vi "Load Firmware Data.vi"(8 "Error In":errorcluster, 9 "Device Type":u16(ring) items=["chipKIT Uno32", "chipKIT uC32", "chipKIT Max32", "chipKIT DP32"], 10 "Device Family":u16(ring) items=["National Instruments", "Digilent", "Arduino"], 11 "Firmware Version":u16(ring) items=["LINX -  Serial / USB", "LINX -  Serial / USB [Debug] "]) -> (0 "Error Out":errorcluster, 2 "Firmware Interface":T1, 3 "Firmware ReadMe":string)   [LabVIEW 2013, in "LVH-LINX.lvlib"]
doc: "Load specified firmware readme."
uses:
  <vilib>/LabVIEW Hacker/LINX/LVH-LINX.lvlib
  <vilib>/LabVIEW Hacker/LINX/Private/Device/Type Defs/Firmware Interface.ctl
panel:
  in  "Device Family":u16(ring) items=["National Instruments", "Digilent", "Arduino"]
  in  "Device Type":u16(ring) items=["chipKIT Uno32", "chipKIT uC32", "chipKIT Max32", "chipKIT DP32"]
  in  "Firmware Version":u16(ring) items=["LINX -  Serial / USB", "LINX -  Serial / USB [Debug] "]
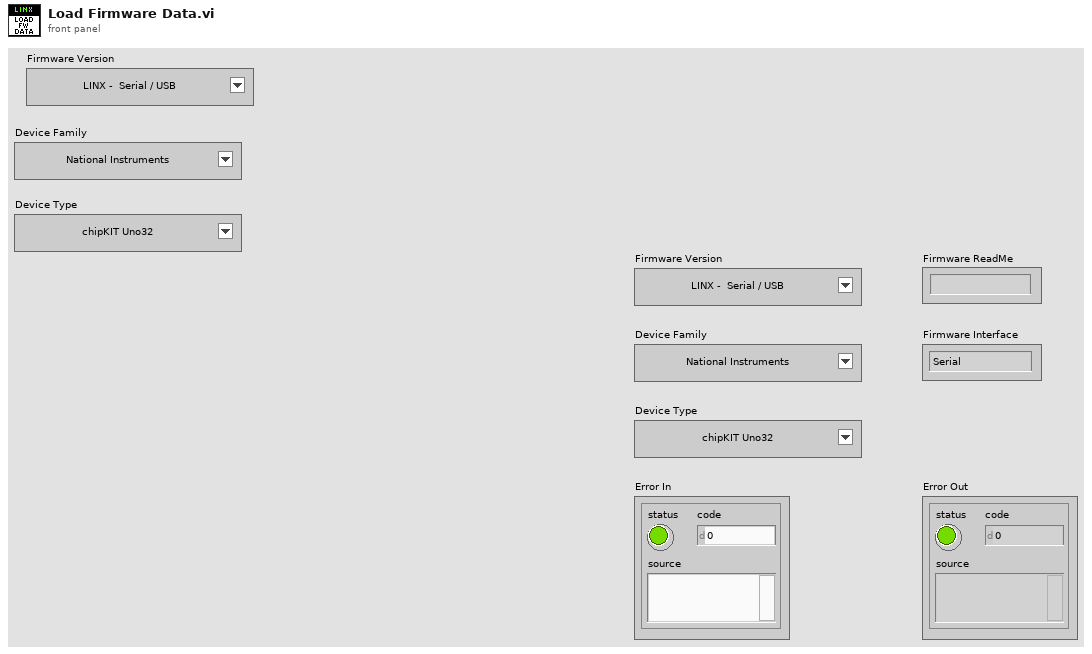
[diagram p1: front panel]
types:
  T1 = typedef "LVH-LINX.lvlib/Firmware Interface.ctl" = enum32{"Serial ", "Ethernet", "WIFI"}
  T2 = typedef "LVH-LINX.lvlib/Generic Device.ctl" = cluster{"DI Channels":u8[], "DO Channels":u8[], "AI":u8[], "AO":u8[], "PWM":u8[], "QE":u8[], "UART":u8[], "I2C 2":u8[], "SPI":u8[], "CAN":u8[], "AI Ref (V)":dbl, "Firmware Program Interfaces":enum16{"N/A", "Serial / USB", "USB", "TCP"}[], "Firmware Versions":T3[], "Name":string, "AO Resolution (Bits)":u8, "AO Ref (V)":dbl}
  T3 = typedef "LVH-LINX.lvlib/Firmware Version.ctl" = cluster{"Name":string, "Relative Path":string, "Firmware Interface":T1}
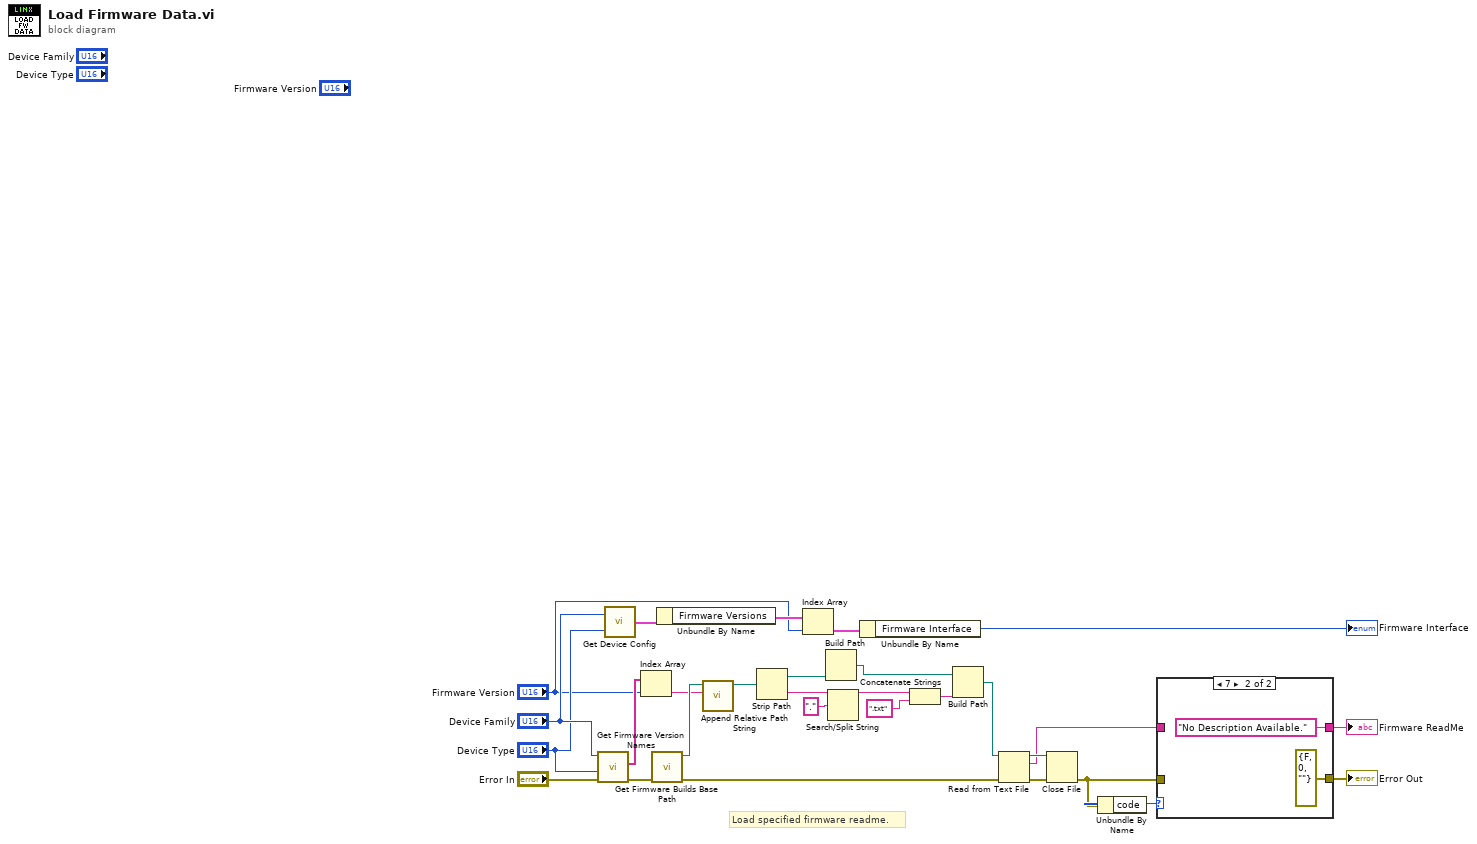
[diagram p0: block diagram]
diagram:
  # "Load specified firmware readme."
  n1 = call <vilib>:"Get Firmware Version Names.vi"("Error In"="Error In", "Device ID"="Device Type", "Device Family"="Device Family") -> ("Error Out"=w28:errorcluster, "Firmware Version Relative Path"=w29:string[])  [unwired: 6 in, 1 out]
  n2 = call <vilib>:"Get Device Config.vi"("Device ID"="Device Type", "Device Family"="Device Family") -> ("Device Config"=w5:T2)
  n3 = Index Array(array=w29, index="Firmware Version") -> (element=w26:string)
  n4 = call <vilib>:"Get Firmware Builds Base Path.vi"("Error In"=w28) -> ("Error Out"=w14:errorcluster, "Firmware Builds Base Path"=w27:path)  [unwired: 9 in]
  n5 = Unbundle By Name(w5) -> ("Firmware Versions"=w4:T3[])
  n6 = call <vilib>:"Append Relative Path String.vi"("Relative Path"=w26, "Base Path"=w27) -> ("Absolute Path"=w18:path)  [unwired: 8 in, 1 out]
  n7 = Strip Path(path=w18) -> (stripped path=w21:path, name=w25:string)
  n8 = Index Array(array=w4, index="Firmware Version") -> (element=w2:T3)
  n9 = Build Path(name or relative path=w21) -> (appended path=w20:path)  [unwired: 1 in]
  n10 = Search/Split String(string=w25, search string/char (-)=".") -> (substring before match=w23:string)  [unwired: 1 in, 2 out]
  n11 = Unbundle By Name(w2) -> ("Firmware Interface"=→"Firmware Interface":T1)
  n12 = Concatenate Strings(w23, ".txt" ("string")) -> (w19:string)
  n13 = Build Path(base path=w20, name or relative path=w19) -> (appended path=w15:path)
  n14 = Read from Text File(file (use dialog)=w15, error in=w14) -> (refnum out=w16:refnum<file>, text=w8:string, error out=w17:errorcluster)  [unwired: 2 in, 1 out]
  n15 = Close File(refnum=w16, error in=w17) -> (error out=w11:errorcluster)  [unwired: 1 out]
  n16 = Unbundle By Name(w11) -> ("code"=w12:i32)
  n17 = case shown="7" w12 {
    tunnel: w11 -> [w30 _]
    tunnel: [w30 errorcluster {"status"=FALSE, "code"=0, "source"=""} ("error out")] -> w10
    tunnel: [w31 "No Description Available."] -> w9
    tunnel: w8 -> [w31 _]
    frame 0, Default {
    }
    frame 7 {
    }
  }
  "Error Out" <- w10
  "Firmware ReadMe" <- w9
